vi "Add Remote Terminal.vi"(8 "error in":errorcluster, 9 "Remote Terminal Config":T1={"rtAddress"=0, "rtMode"=0, "initialSwd"=[0, 0], "noBuild"=FALSE, "autoBusy"=FALSE, "dynamicBC"=FALSE, "clearSwdImmediate"=FALSE, "busEnable"=2, "dataWipe"=0, "syncMode"=0, "responseMode"=1, "responseTime"=9.0} {"responseMode" items=["Selective", "All"]; "syncMode" items=["Zeroes", "Item123", "CWD", "None"]; "dataWipe" items=["A", "B", "AB", "None"]; "busEnable" items=["A", "B", "AB", "None"]; "rtMode" items=["Simulate", "Monitor", "Disable"]}, 10 "name":string, 11 "1553channel ref in":refnum<k24>) -> (0 "error out":errorcluster, 2 "new remoteTerminal":refnum<k24>, 3 "1553channel ref out":refnum<k24>)   [LabVIEW 2020, in "Ballard_1553_Hardware_ni.lvlib"]
uses:
  Ballard_1553_Hardware_ni.lvlib
  C:/Users/Administrator/Desktop/GIT/Ballard-MIL-STD-1553-Custom-Device/Source/System Explorer/SubVIs/Parse XML Ballard/1.2/BTIXML_SerDes.dll
  Ballard-MIL-STD-1553-Custom-Device/Source/System Explorer/SubVIs/Parse XML Ballard/1.2/BTIXML_SerDes.dll
  _typedefs/RemoteTerminal_type.ctl
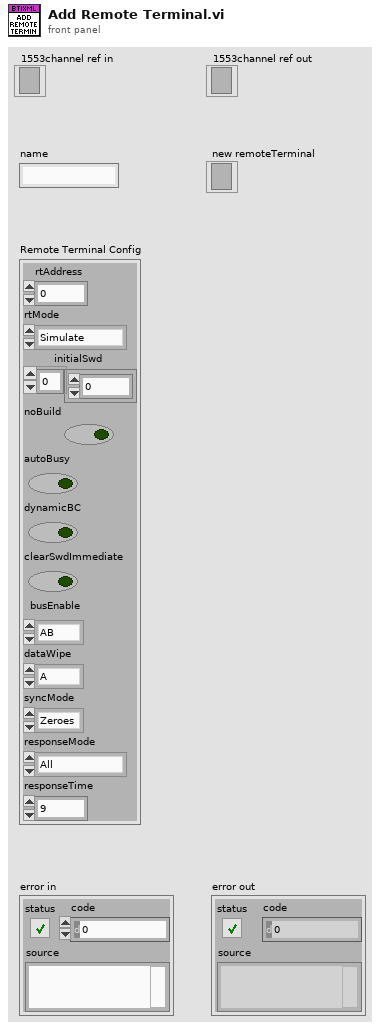
[diagram p1: front panel]
types:
  T1 = typedef "Ballard_1553_Hardware_ni.lvlib/RemoteTerminal_type.ctl" = cluster{"rtAddress":i8, "rtMode":i32, "initialSwd":u8[], "noBuild":bool, "autoBusy":bool, "dynamicBC":bool, "clearSwdImmediate":bool, "busEnable":i32, "dataWipe":i32, "syncMode":i32, "responseMode":i32, "responseTime":dbl}
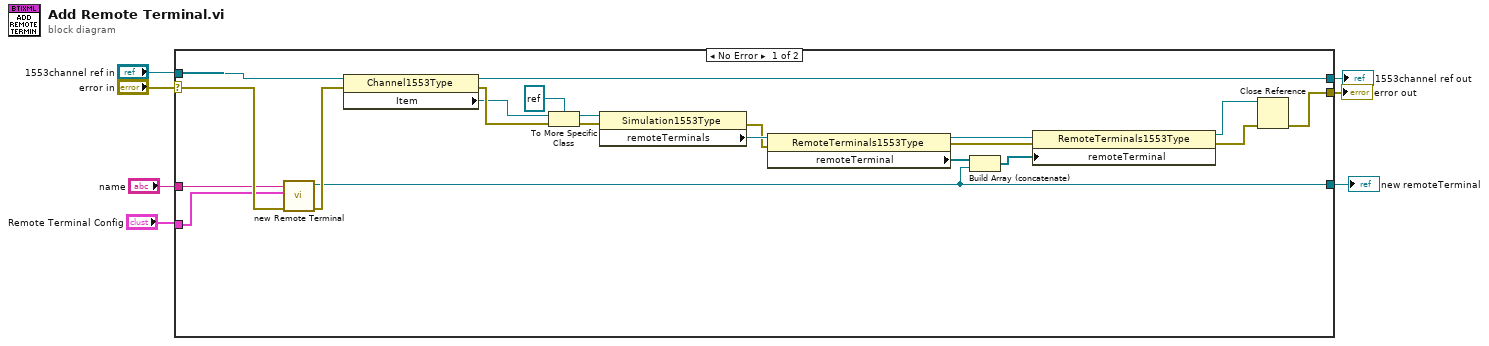
[diagram p0: block diagram]
diagram:
  n1 = case shown="No Error" "error in" {
    selector: "error in" -> [w10 w29]
    tunnel: [w21 w29] -> w7
    tunnel: [w28 w30] -> w6
    tunnel: "1553channel ref in" -> [w27 w30]
    tunnel: [w11 _] -> w3
    tunnel: "name" -> [w9 _]
    tunnel: "Remote Terminal Config" -> [w8 _]
    frame No Error {
      n2 = call "new Remote Terminal.vi"("error in"=w10, "Remote Terminal Config"=w8, "name"=w9) -> ("error out"=w13:errorcluster, "remoteTerminal out"=w11:refnum<k24>)  [unwired: 7 in]
      n3 = property class="Channel1553Type"(reference=w27, error in=w13) -> (reference out=w28:refnum<k24>, error out=w26:errorcluster, "Item"=w25:refnum<k24>)
      n4 = To More Specific Class(target class=refnum<k24> refnum, reference=w25, error in=w26) -> (specific class reference=w23:refnum<k24>, error out=w22:errorcluster)
      n5 = property class="Simulation1553Type"(reference=w23, error in=w22) -> (error out=w17:errorcluster, "remoteTerminals"=w18:refnum<k24>)  [unwired: 1 out]
      n6 = property class="RemoteTerminals1553Type"(reference=w18, error in=w17) -> (reference out=w15:refnum<k24>, error out=w14:errorcluster, "remoteTerminal"=w16:refnum<k24>[])
      n7 = Build Array (concatenate)(w16, w11) -> (w12:refnum<k24>[])
      n8 = property class="RemoteTerminals1553Type"(reference=w15, error in=w14, "remoteTerminal"=w12) -> (reference out=w19:refnum<k24>, error out=w20:errorcluster)
      n9 = Close Reference(reference=w19, error in (no error)=w20) -> (error out=w21:errorcluster)
    }
    frame Error {
    }
  }
  "error out" <- w7
  "1553channel ref out" <- w6
  "new remoteTerminal" <- w3
